vi "Write FRU.vi"(0 "device reference in":T2, 1 "FRU Type":T4, 5 "i2c configuration in":T3, 7 "CSV Path":path, 9 "Unique FRU Input":T1, 11 "error in (no error)":errorcluster, 12 "Write Delay Between Pages (ms)":u32=4) -> (4 "device reference out":T2, 6 "i2c configuration out":T3, 8 "Data Bytes Written":u8[](array[numeric]) format="%02x", 14 "PASS":bool, 15 "error out":errorcluster)   [LabVIEW 2025]
uses:
  Type Definitions/FRU Type.ctl
  <vilib>/ni845x/ni845x.llb/ni845xI2cConfiguration.ctl
  <vilib>/ni845x/ni845x.llb/ni845xControl.ctl
  Type Definitions/Unique FRU Input.ctl
  Type Definitions/I2C Data Address Cluster.ctl
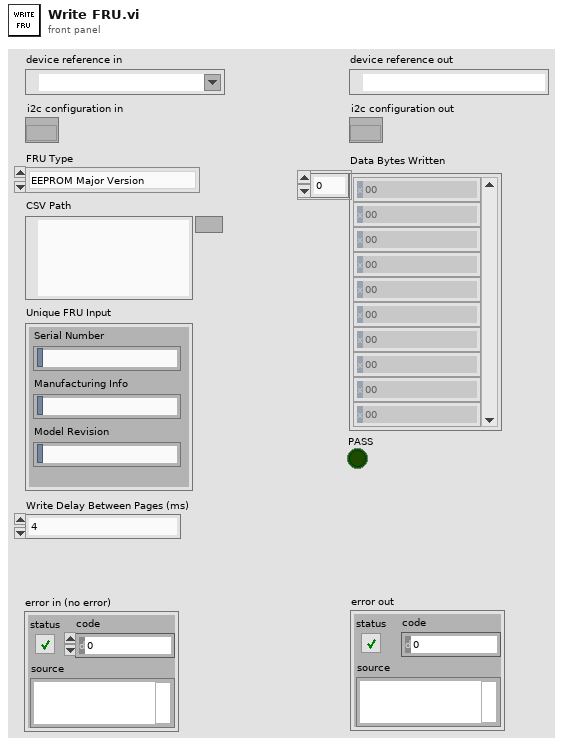
[diagram p1: front panel]
types:
  T1 = typedef "Unique FRU Input.ctl" = cluster{"Serial Number":string, "Manufacturing Info":string, "Model Revision":string}
  T2 = typedef "ni845xControl.ctl" = refnum<k21>
  T3 = typedef "ni845xI2cConfiguration.ctl" = refnum<k20>
  T4 = typedef "FRU Type.ctl" = enum16{"EEPROM Major Version", "EEPROM Minor Version", "nInitialized", "nWriteProtect", "Product Name", "Serial Number", "Manufacturing Info", "Manufacturer Name", "Model Revision", "FW Major Rev", "MCU FW Minor Rev", "Lifetime Turn On Time", "Alarm Enable Flags", "Temperature High", "Battery Charge Low", "Battery Runtime Low", "User System Name", "User Device Name", "Battery Type", "Temperature Unit", "Configuration Flags", "PC Shutdown_Enable/Disable", "Scheduled Shutdown", "PC Shutdown Delay Count_Enable/Disable", "Restart Period", "Event Buffer Length", "Event Write Index", "Event Read Index", "Ambient Temp C.C 0", "Ambient Temp C.C 1", "BEM FET Temp C.C 0", "BEM FET Temp C.C 1", "Flyback TRF Temp C.C 0", "Flyback TRF Temp C.C 1", "Event Data"}
  T5 = typedef "I2C Data Address Cluster.ctl" = cluster{"Data Address Endianness":bool, " Data Address Width":enum16{"1 Byte", "2 Byte"}}
  T6 = typedef "I2C Data Cluster.ctl" = cluster{"Address Byte":u16, "Number of Bytes":u32, "Page Size in Bytes":u32, "Data Byte":u8[], "Write Delay Between Pages (ms)":u32}
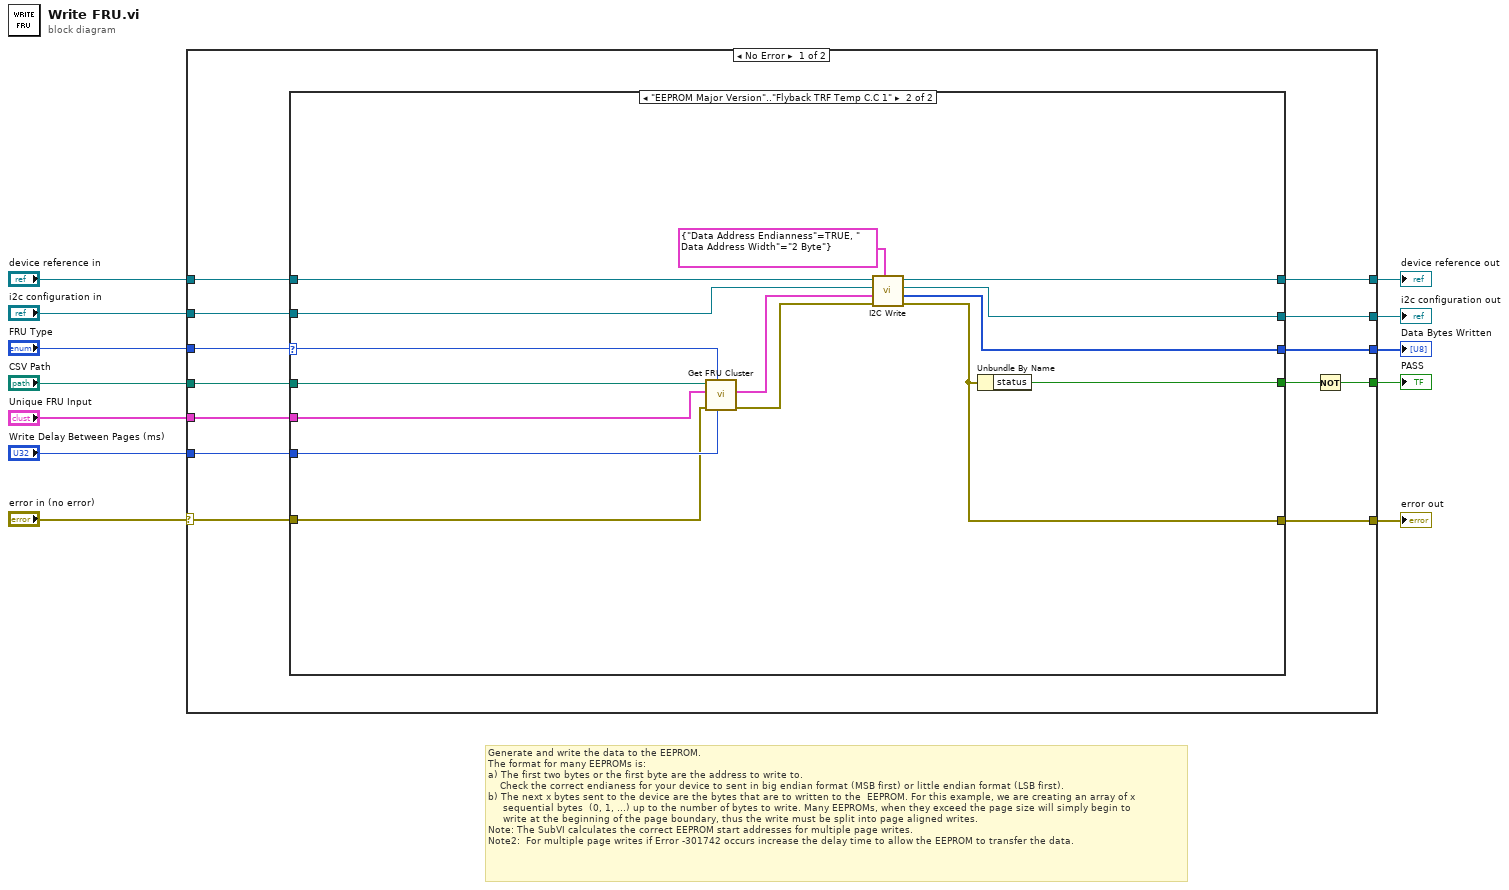
[diagram p0: block diagram]
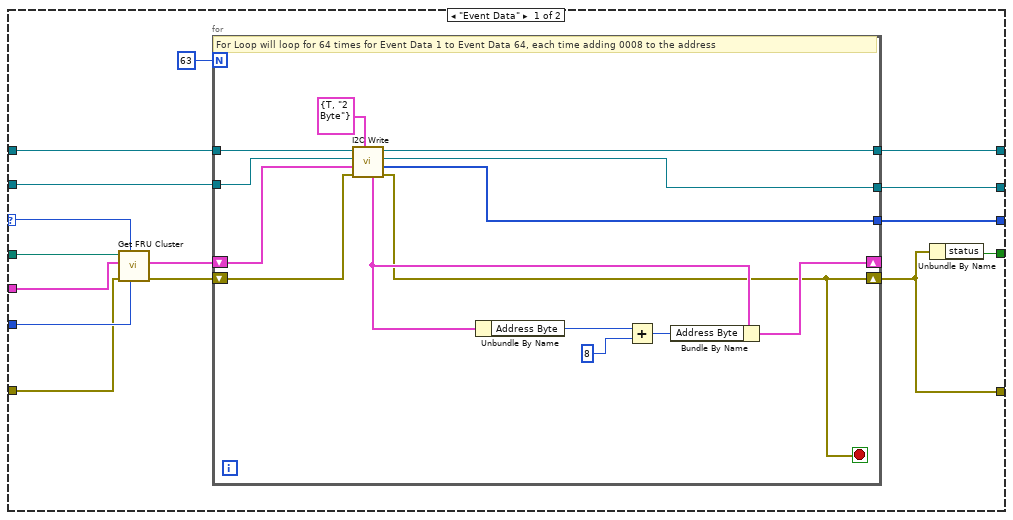
[diagram p2: hidden frame]
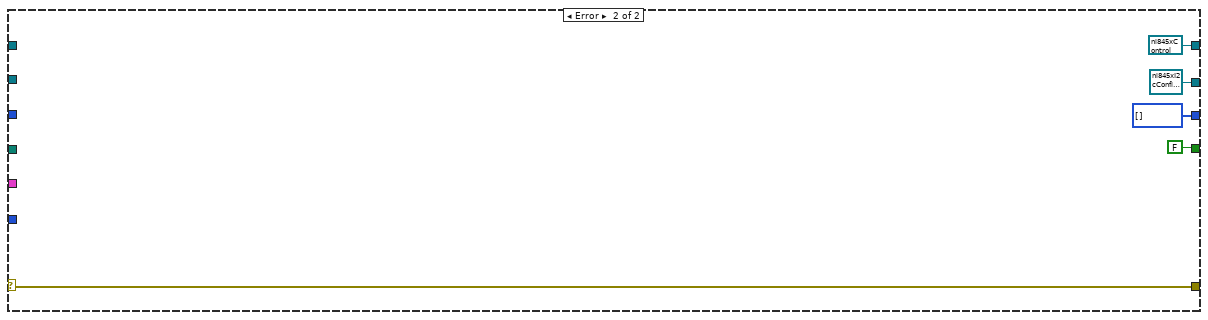
[diagram p3: hidden frame]
diagram:
  # "Generate and write the data to the EEPROM. \nThe format for many EEPROMs is:\na) The first two bytes or the first byte are the address to write to. \n    Check the correct endianess for your device to sent in big endian format (MSB first) or little endian format (LSB first).\nb) The next x bytes sent to the device are the bytes that are to written to the  EEPROM. For this example, we are creating an array of x\n     sequential bytes  (0, 1, ...) up to the number of bytes to write. Many EEPROMs, when they exceed the page size will simply begin to\n     write at the beginning of the page boundary, thus the write must be split into page aligned writes.\nNote: The SubVI calculates the correct EEPROM start addresses for multiple page writes.\nNote2:  For multiple page writes if Error -301742 occurs increase the delay time to allow the EEPROM to transfer the data."
  n1 = case shown="No Error" "error in (no error)" {
    selector: "error in (no error)" -> [w14 w70]
    tunnel: [w17 w70] -> w12
    tunnel: "FRU Type" -> [w13 _]
    tunnel: "i2c configuration in" -> [w20 _]
    tunnel: [w18 T3 refnum ("i2c configuration out")] -> w9
    tunnel: "device reference in" -> [w21 _]
    tunnel: [w19 T2 refnum ("device reference out")] -> w7
    tunnel: [w22 FALSE ("status")] -> w6
    tunnel: "CSV Path" -> [w25 _]
    tunnel: "Unique FRU Input" -> [w24 _]
    tunnel: [w16 u8[] [] ("Data Bytes Written")] -> w3
    tunnel: "Write Delay Between Pages (ms)" -> [w15 _]
    frame No Error {
      n2 = case shown="\"EEPROM Major Version\"..\"Flyback TRF Temp C.C 1\"" w13 {
        selector: w13 -> [w28 w55]
        tunnel: w25 -> [w40 w69]
        tunnel: w24 -> [w39 w68]
        tunnel: [w38 w67] -> w23
        tunnel: w21 -> [w37 w65]
        tunnel: w20 -> [w36 w64]
        tunnel: [w34 w62] -> w19
        tunnel: [w33 w61] -> w18
        tunnel: [w32 w60] -> w17
        tunnel: [w31 w59] -> w16
        tunnel: w15 -> [w30 w57]
        tunnel: w14 -> [w29 w56]
        frame "Event Data" {
          n3 = call "Get FRU Cluster.vi"("Write Delay Between Pages (ms)"=w30, "FRU Type"=w28, "error in (no error)"=w29, "Unique FRU Input"=w39, "CSV Path"=w40) -> ("error out"=w35:errorcluster, "FRU Cluster"=w26:T6)  [unwired: 5 in]
          n4 = for {
            N: 63 -> [_]
            tunnel: [w49] -> w31
            shift-right: [w41] -> w32
            shift-left: w35 -> [w52]
            tunnel: w37 -> [w54]
            tunnel: [w51] -> w34
            tunnel: w36 -> [w53]
            tunnel: [w50] -> w33
            shift-right: [w42] -> _
            shift-left: w26 -> [w46]
            stop <- w41 stop-if-true
            # "For Loop will loop for 64 times for Event Data 1 to Event Data 64, each time adding 0008 to the address"
            n5 = call "I2C Write.vi"("I2C Data Address Cluster"=T5 {"Data Address Endianness"=TRUE, " Data Address Width"=enum."2 Byte"}, "error in (no error)"=w52, "I2C Data Cluster"=w46, "i2c configuration in"=w53, "device reference in"=w54) -> ("error out"=w41:errorcluster, "Data Bytes Written"=w49:u8[], "i2c configuration out"=w50:T3, "device reference out"=w51:T2, "I2C Data Cluster Out"=w47:T6)  [unwired: 2 in]
            n6 = Unbundle By Name(w47) -> ("Address Byte"=w45:u16)
            n7 = Add(x=w45, y=u16 8) -> (x+y=w43:u16)
            n8 = Bundle By Name(cluster=w47, "Address Byte"=w43) -> (w42:T6)
          }
          n9 = Unbundle By Name(w32) -> ("status"=w38:bool)
        }
        frame "EEPROM Major Version".."Flyback TRF Temp C.C 1" {
          n10 = call "Get FRU Cluster.vi"("Write Delay Between Pages (ms)"=w57, "FRU Type"=w55, "error in (no error)"=w56, "Unique FRU Input"=w68, "CSV Path"=w69) -> ("error out"=w63:errorcluster, "FRU Cluster"=w66:T6)  [unwired: 5 in]
          n11 = call "I2C Write.vi"("I2C Data Address Cluster"=T5 {"Data Address Endianness"=TRUE, " Data Address Width"=enum."2 Byte"}, "error in (no error)"=w63, "I2C Data Cluster"=w66, "i2c configuration in"=w64, "device reference in"=w65) -> ("error out"=w60:errorcluster, "Data Bytes Written"=w59:u8[], "i2c configuration out"=w61:T3, "device reference out"=w62:T2)  [unwired: 2 in, 1 out]
          n12 = Unbundle By Name(w60) -> ("status"=w67:bool)
        }
      }
      n13 = Not(x=w23) -> (.not. x?=w22:bool)
    }
    frame Error {
    }
  }
  "error out" <- w12
  "i2c configuration out" <- w9
  "device reference out" <- w7
  "PASS" <- w6
  "Data Bytes Written" <- w3
